vi "Inspect.vi"(9 "Msg":refnum<class "Msg.lvclass">, 10 "Within Msg Set":bool, 11 "Core Actor in":refnum<class "Core Actor.lvclass">) -> (2 "Inspect Proceed":bool=TRUE, 3 "Core Actor out":refnum<class "Core Actor.lvclass">)   [LabVIEW 2025, in "jettl.lvlib" / "Core Actor.lvlib" / "Core Actor.lvclass"]
uses:
  Core Actor.lvclass
  Msg/Msg.lvclass
  Core Actor.lvclass/Core Actor.ctl
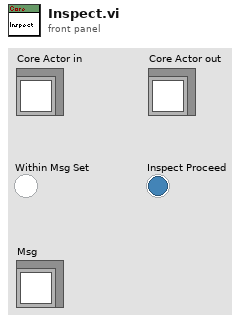
[diagram p1: front panel]
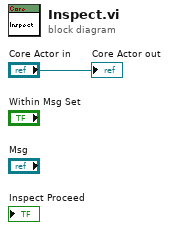
[diagram p0: block diagram]
diagram:
  "Core Actor out" <- "Core Actor in"
